vi "End-processing.vi"(5 "Processing?":refnum<notifier>, 7 "Acquiring?":refnum<notifier>, 8 "error in":errorcluster, 11 "Buffers in":refnum<class "CV-Buffers.lvclass">) -> (0 "error IO":errorcluster, 2 "Continue processing?":bool, 3 "Buffers":refnum<class "CV-Buffers.lvclass">)   [LabVIEW 2013, in "CameraVision.lvlib" / "CV-Main.lvclass"]
uses:
  CV-Main.lvclass
  Buffers/CV-Buffers.lvclass
  Buffers/CV-Buffers.lvclass/CV-Buffers.ctl
  Buffers/Read Processing buffer.vi
  UI/CV-UI.lvclass
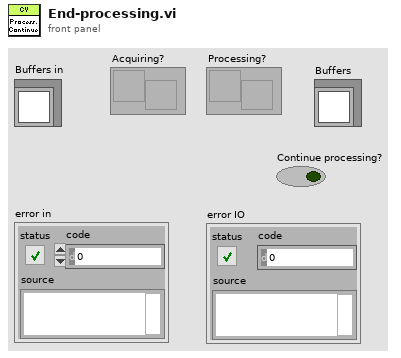
[diagram p1: front panel]
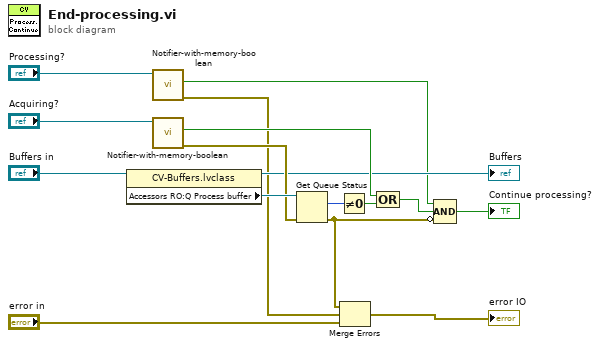
[diagram p0: block diagram]
diagram:
  n1 = property class="CV-Buffers.lvclass"(reference="Buffers in") -> (reference out=→"Buffers":refnum<class "CV-Buffers.lvclass">, "Accessors RO:Q Process buffer"=w14:refnum<queue>)  [unwired: 1 in, 1 out]
  n2 = call "Notifier-with-memory-boolean.vi"("Notifier in"="Processing?") -> ("error IO"=w2:errorcluster, "Notification"=w1:bool)  [unwired: 9 in]
  n3 = call "Notifier-with-memory-boolean.vi"("Notifier in"="Acquiring?") -> ("error IO"=w10:errorcluster, "Notification"=w11:bool)  [unwired: 9 in]
  n4 = Get Queue Status(queue=w14, error in (no error)=w10) -> (# pending remove=w13:i32, error out=w8:errorcluster)  [unwired: 1 in, 6 out]
  n5 = Not Equal To 0?(x=w13) -> (x != 0?=w12:bool)
  n6 = Merge Errors(w8, w2, "error in") -> (→"error IO":errorcluster)
  n7 = Compound Arithmetic op=OR(w11, w12) -> (w9:bool)
  n8 = Compound Arithmetic op=AND(w1, w9, invert w8) -> (→"Continue processing?":bool)
